vi "Cal Debug.vi"() -> ()   [LabVIEW 2011, in "Debug Variable Library.lvlib"]
uses:
  Debug Variable Library.lvlib
  RT Config Data.ctl
  TC Channel Config Data.ctl
  TC Selector.ctl
  TC Unit Selector.ctl
  RT TC Update State.ctl
  Simulated Thermocouple Custom Device.lvlib
panel:
  in  "stop":bool
  out "Cal Valid?":bool
  out "Percent Error":dbl[](array[numeric])
  out "Voltages to Output":dbl[](array[numeric])
  in  "simTC Channels":dbl[](array[numeric])
  in  "Cal Channels":dbl[](array[numeric])
  in  "TC Update State":T1
  in  "RT Configuration Data":T2 {"Cal Types" items=["J", "K", "T", "E", "N", "B", "R", "S"]; "Temperature Units" items=["Celcius", "Fahrenheit", "Kelvin", "Rankine"]; "TC Channel Config"."Temperature Units" items=["Celcius", "Fahrenheit", "Kelvin", "Rankine", "Volts"]; "TC Channel Config"."Thermocouple Type" items=["J", "K", "T", "E", "N", "B", "R", "S", "Raw Voltage"]}
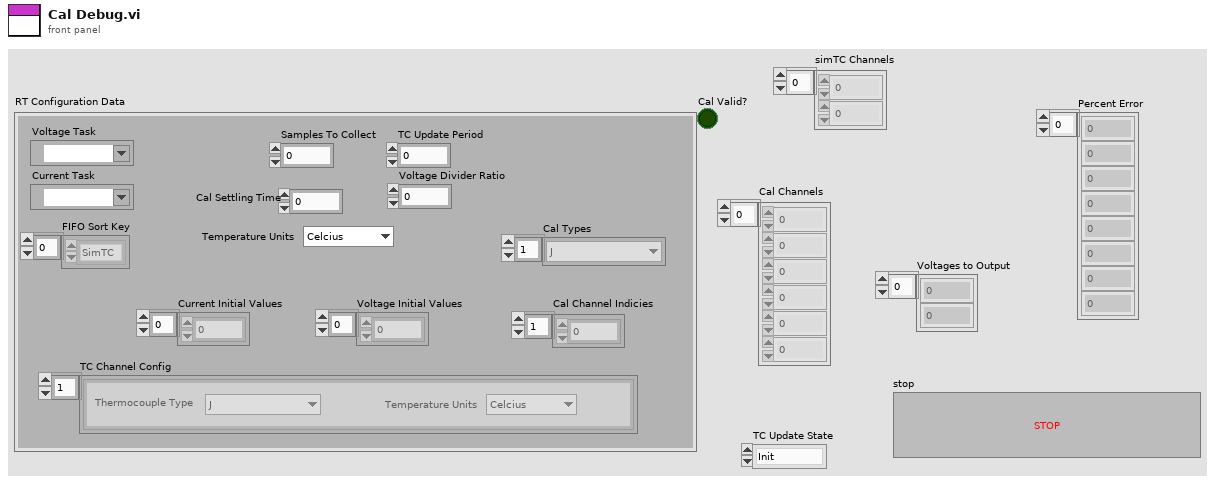
[diagram p1: front panel]
types:
  T1 = typedef "Simulated Thermocouple Custom Device.lvlib/RT TC Update State.ctl" = enum16{"Init", "Calibrate", "Update", "Idle"}
  T2 = typedef "Simulated Thermocouple Custom Device.lvlib/RT Config Data.ctl" = cluster{"Current Task":refnum<k21>, "Voltage Task":refnum<k21>, "FIFO Sort Key":enum16{"SimTC", "Calibration", "VO", "CO"}[], "Cal Channel Indicies":i32[], "Current Initial Values":dbl[], "Voltage Initial Values":dbl[], "TC Channel Config":T3[], "TC Update Period":dbl, "Voltage Divider Ratio":dbl, "Samples To Collect":dbl, "Temperature Units":T5, "Cal Settling Time":dbl, "Cal Types":T4[]}
  T3 = typedef "Simulated Thermocouple Custom Device.lvlib/TC Channel Config Data.ctl" = cluster{"Thermocouple Type":T4, "Temperature Units":T5}
  T4 = typedef "Simulated Thermocouple Custom Device.lvlib/TC Selector.ctl" = u16
  T5 = typedef "Simulated Thermocouple Custom Device.lvlib/TC Unit Selector.ctl" = u16
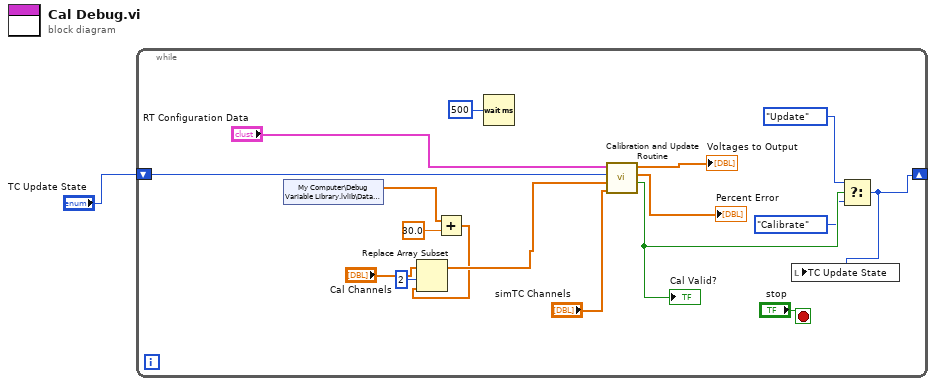
[diagram p0: block diagram]
diagram:
  n1 = while {
    shift-right: [w2] -> _
    shift-left: "TC Update State" -> [w6]
    stop <- "stop" stop-if-true
    n2 = shared-variable "My Computer\\Debug Variable Library.lvlib\\Data Array"() -> (w8:dbl[])  [unwired: 1 in, 1 out]
    n3 = Add(x=w8, y=30.0) -> (x+y=w7:dbl[])
    n4 = Replace Array Subset(array="Cal Channels", new element=w7, index=2) -> (w10:dbl[])
    n5 = Wait (ms)(milliseconds to wait=u32 500) -> ()  [unwired: 1 out]
    n6 = call "Calibration and Update Routine.vi"("simTC Channels"="simTC Channels", "Cal Channels"=w10, "TC Update State"=w6, "RT Configuration Data"="RT Configuration Data") -> ("Cal Valid?"=w5:bool, "Error"=→"Percent Error":dbl[], "Voltages to Output"=→"Voltages to Output":dbl[])  [unwired: 5 in]
    "Cal Valid?" <- w5
    n7 = Select(t=RT_TC_Update_State."Update" ("TC Update State"), s=w5, f=RT_TC_Update_State."Calibrate" ("TC Update State")) -> (s? t:f=w2:T1)
    n8 = local write "TC Update State"(w2) -> ()
  }
